vi "Benchmark Calculate Curve Distance.vi"() -> ()   [LabVIEW 2019]
uses:
  Parse/PathCommands/Point.ctl
  Tool Path.lvclass
  Parse/PathCommands/PathCommands.lvclass
panel:
  out "Array":dbl[](array[numeric])
  out "Points Out":T1[][](array[typedef])
  out "x/y":dbl
  # "scales linearly with number of iterations"
  # "inkscape: 15727.82"
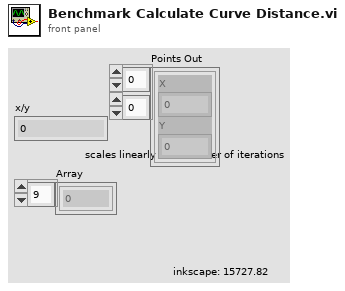
[diagram p1: front panel]
types:
  T1 = typedef "PathCommands.lvclass/Point.ctl" = cluster{"X":dbl, "Y":dbl}
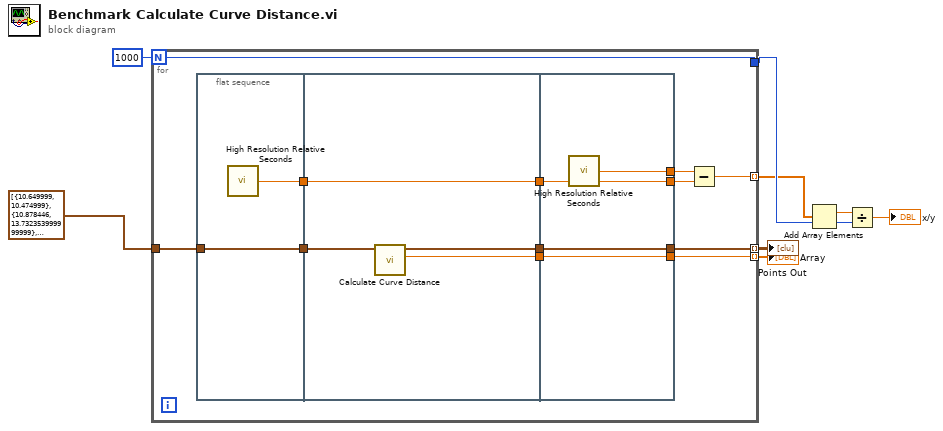
[diagram p0: block diagram]
diagram:
  n1 = for {
    N: 1000 -> [w11]
    tunnel: T1[] [{"X"=10.649999, "Y"=10.474999}, {"X"=10.878446, "Y"=13.732353999999999}, {"X"=13.823540999999999, "Y"=15.099646}, {"X"=14.093748999999999, "Y"=20.668749}] ("Points") -> [w20]
    tunnel: [w13] -> w3 mode=indexing
    tunnel: [w12] -> w5 mode=indexing
    tunnel: [w11] -> w7
    tunnel: [w10] -> w2 mode=indexing
    n2 = flat-sequence {
      tunnel: w20 -> [w21]
      tunnel: [w22] -> w19
      tunnel: [w21] -> w15
      tunnel: w19 -> [w26]
      tunnel: [w26] -> w17
      tunnel: w15 -> [w25]
      tunnel: [w24] -> w14
      tunnel: [w23] -> w9
      tunnel: [w30] -> w18
      tunnel: w17 -> [w29]
      tunnel: [w29] -> w16
      tunnel: w14 -> [w28]
      tunnel: [w28] -> w13
      tunnel: [w27] -> w10
      tunnel: w9 -> [w27]
      frame #0 {
        n3 = call <vilib>:"High Resolution Relative Seconds.vi"() -> ("relative seconds"=w22:dbl)
      }
      frame #1 {
        n4 = call "Calculate Curve Distance.vi"("Points"=w25) -> ("Length"=w23:dbl, "Points Out"=w24:T1[])  [unwired: 8 in, 1 out]
      }
      frame #2 {
        n5 = call <vilib>:"High Resolution Relative Seconds.vi"() -> ("relative seconds"=w30:dbl)
      }
    }
    n6 = Subtract(x=w18, y=w16) -> (x-y=w12:dbl)
  }
  "Points Out" <- w3
  "Array" <- w2
  n7 = Add Array Elements(numeric array=w5) -> (sum=w6:dbl)
  n8 = Divide(x=w6, y=w7) -> (x/y=→"x/y":dbl)
